vi "Read Ai.vi"(0 "FPGA API in":refnum<class "FPGA API Mock.lvclass">, 11 "error in (no error)":errorcluster) -> (4 "FPGA API out":refnum<class "FPGA API Mock.lvclass">, 6 "AI Data":dbl[][](array[numeric]), 8 "Valud Data":bool, 15 "error out":errorcluster)   [LabVIEW 2019, in "FPGA API Mock.lvclass"]
uses:
  FPGA API Mock.lvclass
  FPGA API Mock.lvclass/FPGA API Mock.ctl
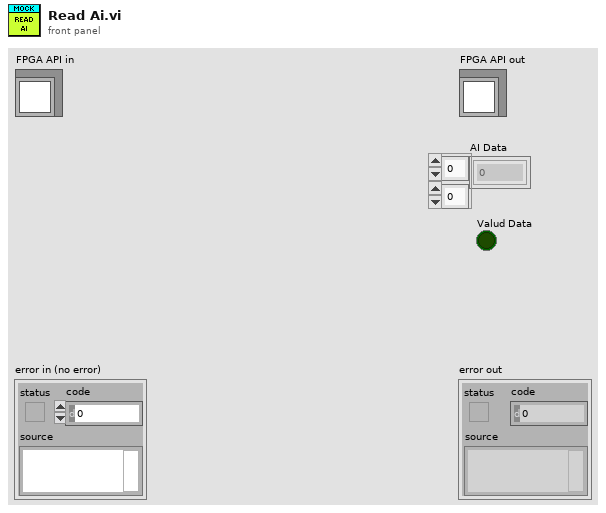
[diagram p1: front panel]
types:
  T1 = typedef "FPGA API Mock.lvclass/Data.ctl" = cluster{"DO":bool[], "DI":bool[], "AI":dbl[], "AO":dbl[]}
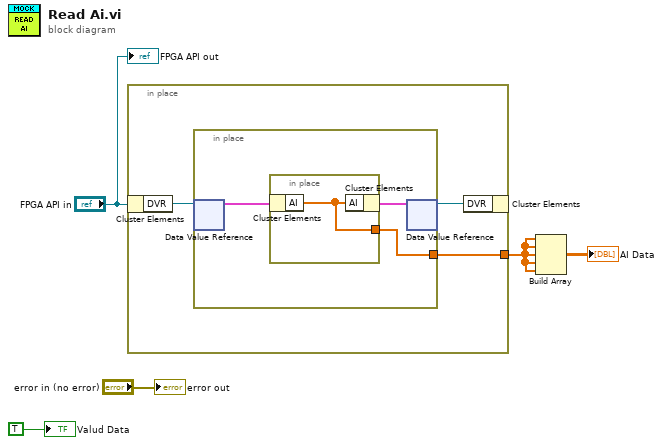
[diagram p0: block diagram]
diagram:
  n1 = in-place {
    in-place-border: [w6] -> w1
    n2 = in-place-cluster #1("FPGA API in") -> ("DVR"=w7:refnum<data-value>)
    n3 = in-place {
      in-place-border: [w9] -> w6
      n4 = in-place-dvr #2(w7) -> (w11:T1)  [unwired: 1 out]
      n5 = in-place {
        in-place-border: [w12] -> w9
        n6 = in-place-cluster #3(w11) -> ("AI"=w12:dbl[])
        n7 = in-place-cluster #3("AI"=w12) -> (w10:T1)
      }
      n8 = in-place-dvr #2(w10) -> (w8:refnum<data-value>)  [unwired: 1 out]
    }
    n9 = in-place-cluster #1("DVR"=w8) -> ()  [unwired: 1 out]
  }
  n10 = Build Array(w1, w1, w1, w1, w1) -> (→"AI Data":dbl[][])
  "error out" <- "error in (no error)"
  "FPGA API out" <- "FPGA API in"
  "Valud Data" <- TRUE ("Valud Data")
